vi "总磷启动参数对话框.vi"() -> (2 "确认":bool, 3 "元素":cluster{"命令":string, "data":variant})   [LabVIEW 2016, in "斯坦道总磷.lvlib"]
panel:
  in  "取消":bool
  in  "确定":bool
  in  "测量间隔":u16
  in  "模式设置":T1(ring)
  in  "量程切换":enum32{"H", "L", "AUTO"}(radio)=enum."AUTO"
  in  "站号":u16(ring)=1 items=["总磷"=1, "总氮"=2]
  in  "控制命令":T2(ring)
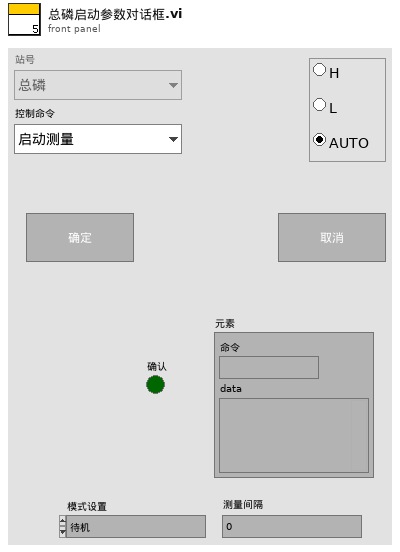
[diagram p1: front panel]
types:
  T1 = enum16{"待机", "连续模式", "周期模式", "定点模式", "受控模式", "手动模式"}
  T2 = enum16{"启动测量", "标样核查", "零点核查", "跨度核查", "空白测试", "平行样测试", "加标回收", "空白校准", "标样校准", "初始化（清洗）", "停止测试", "仪器重启", "校时", "模式设置", "测量间隔设置"}
  T3 = cluster{"站号":u16, "量程切换":enum32{"H", "L", "AUTO"}, "控制命令":enum16{"启动测量", "标样核查", "零点核查", "跨度核查", "空白测试", "平行样测试", "加标回收", "空白校准", "标样校准", "初始化（清洗）", "停止测试", "仪器重启", "校时", "模式设置", "测量间隔设置", "盲样测试"}, "模式设置":enum16{"待机", "连续模式", "周期模式", "定点模式", "受控模式", "手动模式"}, "测量间隔":u16}
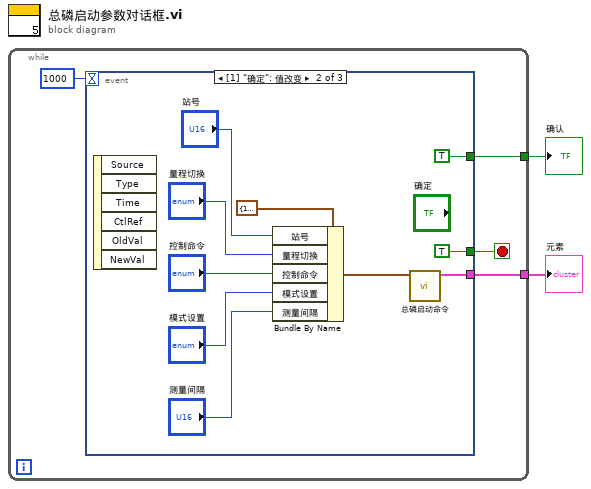
[diagram p0: block diagram]
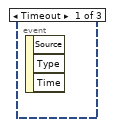
[diagram p2: hidden frame]
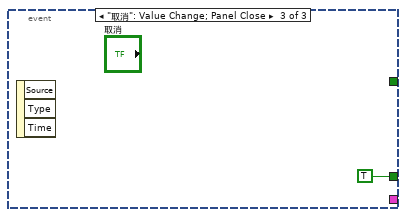
[diagram p3: hidden frame]
diagram:
  n1 = while {
    tunnel: [w4] -> w2
    tunnel: [w3] -> w1
    stop <- w6 stop-if-true
    n2 = event shown="[1] \"确定\": 值改变" {
      selector: _ -> [_ _ _]
      dyn-events: _ -> [_ _ _]
      timeout: 1000 -> [_ _ _]
      tunnel: [_ TRUE TRUE] -> w6
      tunnel: [_ TRUE _] -> w4
      tunnel: [_ w14 _] -> w3
      event Timeout {
        n3 = event-data() -> ()  [unwired: 1 in, 3 out]
      }
      event "确定": Value Change {
        n4 = event-data() -> ()  [unwired: 1 in, 6 out]
        n5 = Bundle By Name(cluster=T3 {"站号"=1, "量程切换"=enum."AUTO", "控制命令"=enum."启动测量", "模式设置"=enum."待机", "测量间隔"=0} ("参数"), "站号"="站号", "量程切换"="量程切换", "控制命令"="控制命令", "模式设置"="模式设置", "测量间隔"="测量间隔") -> (w12:T3)
        n6 = call "总磷启动命令.vi"("参数"=w12) -> ("启动命令"=w14:cluster{"命令":string, "data":variant})  [unwired: 10 in]
      }
      event "取消": Value Change; Panel Close {
        n7 = event-data() -> ()  [unwired: 1 in, 3 out]
      }
    }
  }
  "元素" <- w1
  "确认" <- w2
